vi "Configure Trigger (I2C - Start,Stop,Missing Ack).vi"(0 "VISA resource name":refnum<visa-resource-name>, 1 "Trigger On (0:Start)":u16(ring) items=["Start", "Stop", "Repeated Start", "Missing ack"], 2 "Addressing Mode (0:7 Bit)":u16(ring) items=["7 Bit", "10 Bit"], 5 "Data Source":T2={"Data Source (0:Channel1)"=0, "Data Threshold (1.2V)"=1.2} {"Data Source (0:Channel1)" items=["Channel1", "Channel2", "Channel3", "Channel4"]}, 7 "Clock Source":T1={"Clock Source (1:Channel2) "=1, "Clock Threshold (1.2V)"=1.2} {"Clock Source (1:Channel2)" items=["Channel1", "Channel2", "Channel3", "Channel4"]}, 9 "Data Direction (0:Either)":u16(ring) items=["Either", "Read", "Write"], 11 "error in (no error)":errorcluster) -> (4 "VISA resource name out":refnum<visa-resource-name>, 15 "error out":errorcluster)   [LabVIEW 2015, in "Tektronix 7000 Series.lvlib"]
doc: "Configures I2C trigger settings for an oscilloscope. A trigger occurs when an Inter-IC Control signal is found. This Vi is configure trigger on Start,RepeatStart,Stop and Missing Ask.\n\n<b>Note:</b>\nOnly DPO7000 series oscilloscopes Support this Trigger."
uses:
  <instrlib>/Tektronix 7000 Series/Tektronix 7000 Series.lvlib
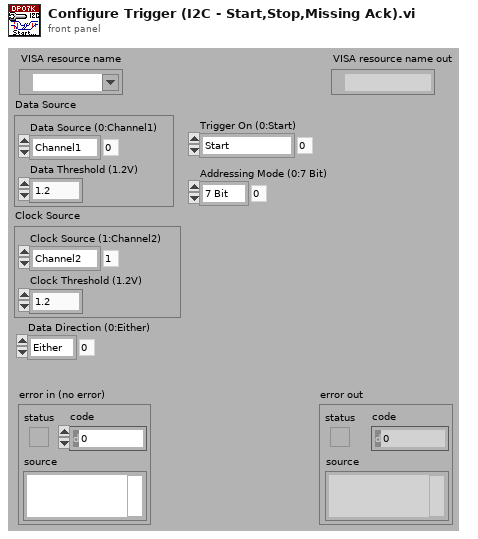
[diagram p1: front panel]
types:
  T1 = cluster{"Clock Source (1:Channel2) ":u16, "Clock Threshold (1.2V)":dbl}
  T2 = cluster{"Data Source (0:Channel1)":u16, "Data Threshold (1.2V)":dbl}
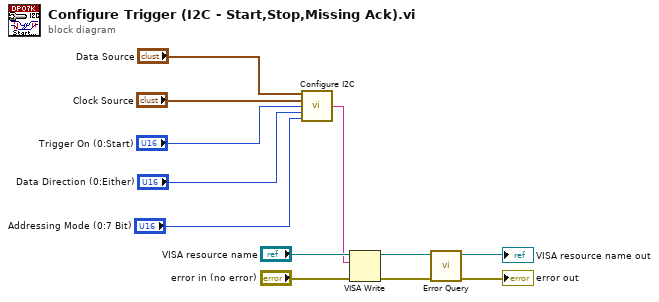
[diagram p0: block diagram]
diagram:
  n1 = call <instrlib>:"Configure I2C.vi"("Data Source"="Data Source", "Clock Source"="Clock Source", "Trigger On (0:Start)"="Trigger On (0:Start)", "Data Direction (0:Either)"="Data Direction (0:Either)", "Addressing Mode (0:7 Bit)"="Addressing Mode (0:7 Bit)") -> ("Output String"=w8:string)  [unwired: 10 in]
  n2 = VISA Write(VISA resource name="VISA resource name", write buffer=w8, error in (no error)="error in (no error)") -> (VISA resource name out=w12:refnum<visa-resource-name>, error out=w11:errorcluster)  [unwired: 1 out]
  n3 = call <instrlib>:"Error Query.vi"("error in (no error)"=w11, "VISA resource name"=w12) -> ("error out"=→"error out":errorcluster, "VISA resource name out"=→"VISA resource name out":refnum<visa-resource-name>)  [unwired: 6 in, 2 out]
